vi "Add VIs and their Protperties to Tree.vi"(6 "File Extension Filters":string[](array[string]), 8 "error in":errorcluster, 11 "Data Tree":refnum<vi>) -> (0 "error out":errorcluster)   [LabVIEW 2013]
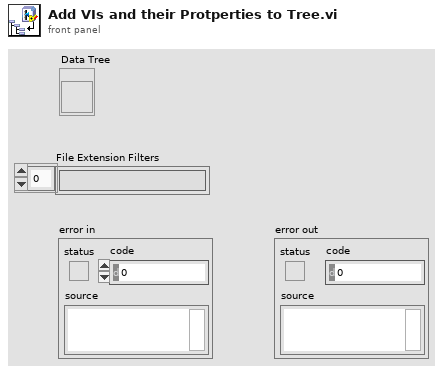
[diagram p1: front panel]
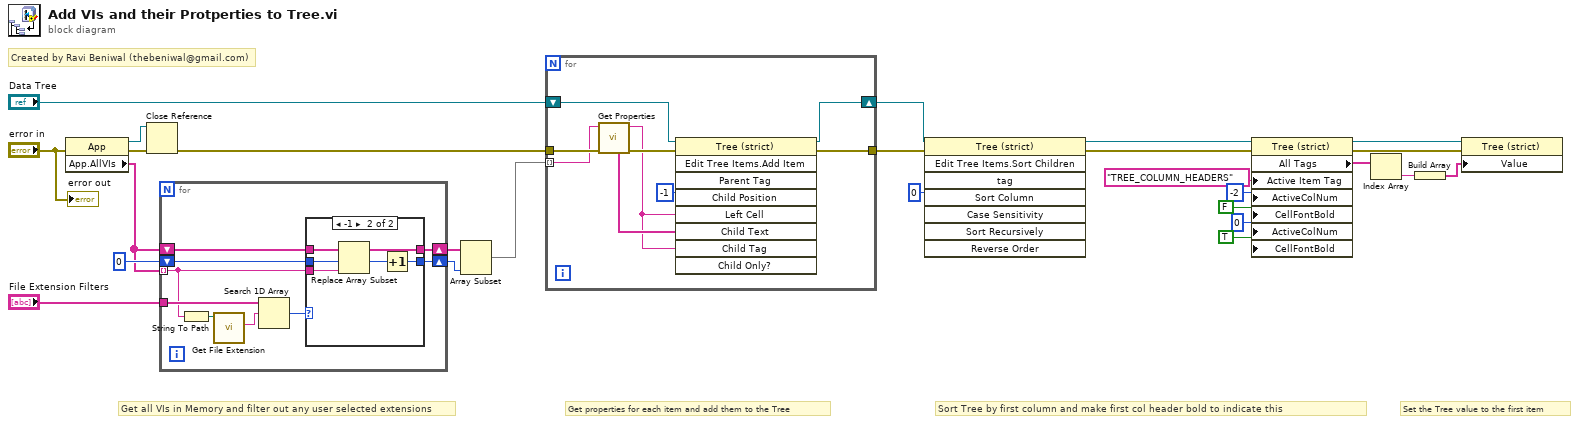
[diagram p0: block diagram]
diagram:
  # "Sort Tree by first column and make first col header bold to indicate this"
  # "Created by Ravi Beniwal (thebeniwal@gmail.com)"
  # "Set the Tree value to the first item"
  # "Get properties for each item and add them to the Tree"
  # "Get all VIs in Memory and filter out any user selected extensions"
  n1 = property class="App"(error in="error in") -> (reference out=w25:refnum<vi>, error out=w26:errorcluster, "App.AllVIs"=w17:string[])  [unwired: 1 in]
  n2 = Close Reference(reference=w25, error in (no error)=w26) -> (error out=w23:errorcluster)
  n3 = for {
    tunnel: w17 -> [w29] mode=indexing
    tunnel: "File Extension Filters" -> [w34]
    shift-right: [w30] -> w19
    shift-left: w17 -> [w31]
    shift-right: [w27] -> w18
    shift-left: 0 -> [w28]
    n4 = String To Path(string=w29) -> (path=w35:path)
    n5 = call <vilib>:"Get File Extension.vi"("file"=w35) -> ("lowercase file extension"=w33:string)  [unwired: 7 in, 3 out]
    n6 = Search 1D Array(1D array=w34, element=w33) -> (index of element=w32:i32)  [unwired: 1 in]
    n7 = case shown="-1" w32 {
      tunnel: w31 -> [w37 w42]
      tunnel: [w37 w41] -> w30
      tunnel: w29 -> [_ w40]
      tunnel: w28 -> [w36 w39]
      tunnel: [w36 w38] -> w27
      frame 0, Default {
      }
      frame -1 {
        n8 = Replace Array Subset(array=w42, new element=w40, index=w39) -> (w41:string[])
        n9 = Increment(x=w39) -> (x+1=w38:i32)
      }
    }
  }
  n10 = Array Subset(array=w19, length=w18) -> (w16:string[])  [unwired: 1 in]
  n11 = for {
    tunnel: w16 -> [w44] mode=indexing
    tunnel: w23 -> [w47]
    tunnel: [w46] -> w13
    shift-right: [w45] -> w10
    shift-left: "Data Tree" -> [w50]
    n12 = call "Get Properties.vi"("error in"=w47, "VI Name"=w44) -> ("error out"=w48:errorcluster, "VI Name Out"=w43:string, "VI Properties"=w49:string[])  [unwired: 5 in, 2 out]
    n13 = invoke on="Invoke Node" class="Tree (strict)" method="Edit Tree Items.Add Item"(reference=w50, error in=w48, "Child Position"=-1, "Left Cell"=w43, "Child Text"=w49, "Child Tag"=w43) -> (reference out=w45:refnum<vi>, error out=w46:errorcluster)  [unwired: 3 in, 7 out]
  }
  n14 = invoke on="Invoke Node" class="Tree (strict)" method="Edit Tree Items.Sort Children"(reference=w10, error in=w13, "Sort Column"=0) -> (reference out=w11:refnum<vi>, error out=w12:errorcluster)  [unwired: 5 in, 6 out]
  n15 = property class="Tree (strict)"(reference=w11, error in=w12, "Active Item Tag"="TREE_COLUMN_HEADERS" ("Active Item:Tag"), "ActiveColNum"=-2 ("Active Cell:Active Column Number"), "CellFontBold"=FALSE ("Active Cell:Cell Font:Bold"), "ActiveColNum"=0 ("Active Cell:Active Column Number"), "CellFontBold"=TRUE ("Active Cell:Cell Font:Bold")) -> (reference out=w7:refnum<vi>, error out=w8:errorcluster, "All Tags"=w9:string[])
  n16 = Index Array(array=w9) -> (element=w6:string)  [unwired: 1 in]
  n17 = Build Array(w6) -> (w15:string[])
  n18 = property class="Tree (strict)"(reference=w7, error in=w8, "Value"=w15) -> ()  [unwired: 2 out]
  "error out" <- "error in"
